vi "respond to response.vi"(7 "last line":u32, 8 "error in (no error)":errorcluster caption="Fehler (Eingang, kein Fehler)", 9 "last response":string, 10 "old Commandlist":string, 11 "Spannungseinbruch Eingang":refnum<class "Spannungseinbruch.lvclass"> caption="DNL_LabVIEW Object in") -> (0 "error out":errorcluster caption="Fehler (Ausgang)", 1 "read again?":bool, 2 "new Commandlist":string, 3 "Spannungseinbruch Ausgang":refnum<class "Spannungseinbruch.lvclass"> caption="DNL_LabVIEW Object out")   [LabVIEW 2013, in "Spannungseinbruch.lvclass"]
uses:
  Spannungseinbruch.lvclass
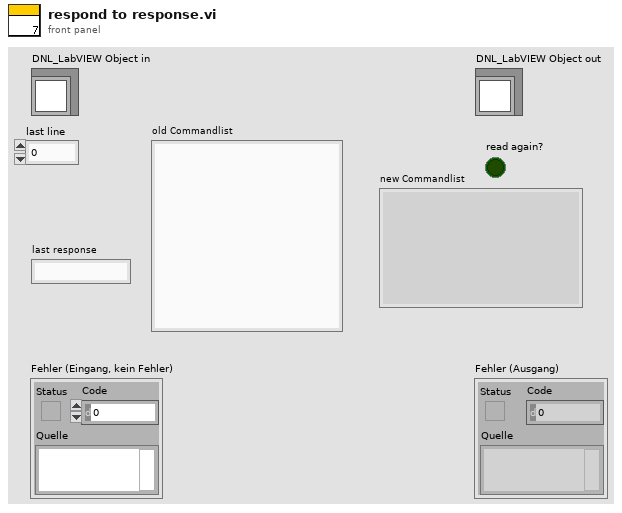
[diagram p1: front panel]
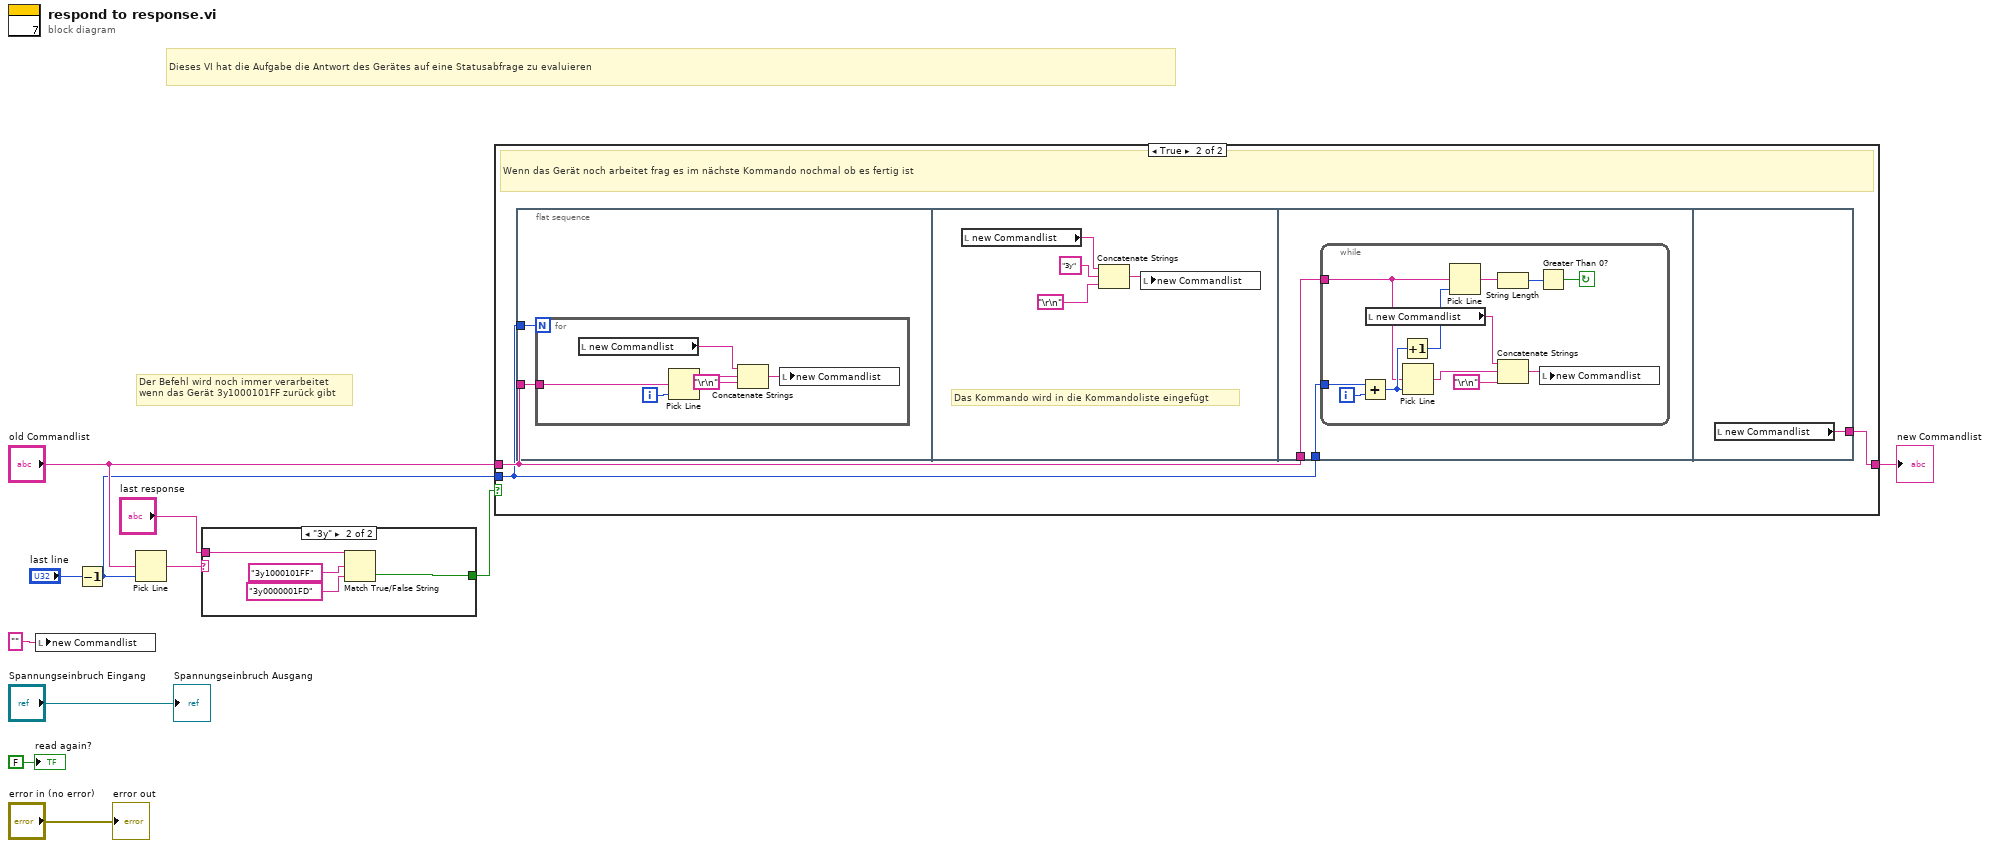
[diagram p0: block diagram]
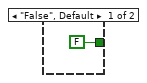
[diagram p3: hidden frame]
diagram:
  # "Dieses VI hat die Aufgabe die Antwort des Gerätes auf eine Statusabfrage zu evaluieren"
  # "Der Befehl wird noch immer verarbeitet\nwenn das Gerät 3y1000101FF zurück gibt"
  n1 = local write "new Commandlist"("" ("new Commandlist")) -> ()
  n2 = Decrement(x="last line") -> (x-1=w1:u32)
  n3 = Pick Line(multi-line string="old Commandlist", line index=w1) -> (output string=w11:string)  [unwired: 1 in]
  n4 = case shown="\"3y\"" w11 {
    tunnel: "last response" -> [_ w16]
    tunnel: [FALSE w13] -> w7
    frame "False", Default {
    }
    frame "3y" {
      n5 = Match True/False String(2:"3y0000001FD" ("regular expression"), 3:"3y1000101FF" ("regular expression"), 4:w16) -> (0:w13:bool)  [unwired: 1 out]
    }
  }
  n6 = case shown="True" w7 {
    tunnel: "old Commandlist" -> [w17 w20]
    tunnel: w1 -> [_ w19]
    tunnel: [w17 w18] -> w6
    frame False {
    }
    frame True {
      # "Wenn das Gerät noch arbeitet frag es im nächste Kommando nochmal ob es fertig ist"
      n7 = flat-sequence {
        tunnel: w19 -> [w22]
        tunnel: w20 -> [w21]
        tunnel: w20 -> [w34]
        tunnel: w19 -> [w33]
        tunnel: [w47] -> w18
        frame #0 {
          n8 = for {
            N: w22 -> [_]
            tunnel: w21 -> [w26]
            i -> [w27]
            n9 = local read "new Commandlist"() -> (w25:string)
            n10 = Pick Line(multi-line string=w26, line index=w27) -> (output string=w24:string)  [unwired: 1 in]
            n11 = Concatenate Strings(w25, w24, "\r\n") -> (w28:string)
            n12 = local write "new Commandlist"(w28) -> ()
          }
        }
        frame #1 {
          # "Das Kommando wird in die Kommandoliste eingefügt"
          n13 = local read "new Commandlist"() -> (w31:string)
          n14 = Concatenate Strings(w31, "3y" ("new Commandlist"), "\r\n") -> (w32:string)
          n15 = local write "new Commandlist"(w32) -> ()
        }
        frame #2 {
          n16 = while {
            tunnel: w34 -> [w42]
            tunnel: w33 -> [w45]
            i -> [w46]
            stop <- w39 continue-if-true
            n17 = Add(x=w45, y=w46) -> (x+y=w44:u32)
            n18 = local read "new Commandlist"() -> (w37:string)
            n19 = Increment(x=w44) -> (x+1=w43:u32)
            n20 = Pick Line(multi-line string=w42, line index=w44) -> (output string=w36:string)  [unwired: 1 in]
            n21 = Pick Line(multi-line string=w42, line index=w43) -> (output string=w41:string)  [unwired: 1 in]
            n22 = String Length(string=w41) -> (length=w40:i32)
            n23 = Concatenate Strings(w37, w36, "\r\n") -> (w38:string)
            n24 = Greater Than 0?(x=w40) -> (x > 0?=w39:bool)
            n25 = local write "new Commandlist"(w38) -> ()
          }
        }
        frame #3 {
          n26 = local read "new Commandlist"() -> (w47:string)
        }
      }
    }
  }
  "new Commandlist" <- w6
  "error out" <- "error in (no error)"
  "Spannungseinbruch Ausgang" <- "Spannungseinbruch Eingang"
  "read again?" <- FALSE ("read again?")
